vi "GetDriverFileName.vi"(11 "input string":string) -> (1 "DriverFileName":string, 2 "数组":string[](array[string]), 3 "子字符串之前":string)   [LabVIEW 2018]
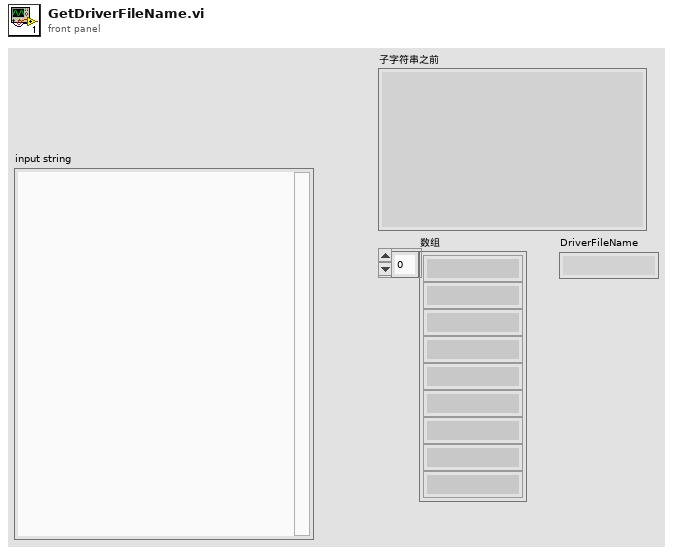
[diagram p1: front panel]
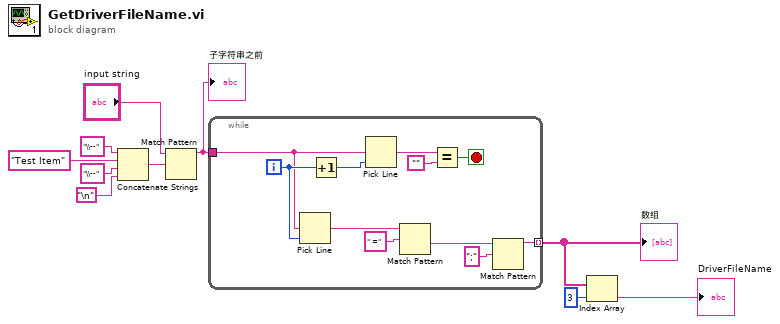
[diagram p0: block diagram]
diagram:
  n1 = Concatenate Strings("\\--" ("regular expression"), "Test Item" ("string"), "\\--" ("string"), "\n") -> (w5:string)
  n2 = Match Pattern(string="input string", regular expression=w5) -> (before substring=w4:string)  [unwired: 4 out]
  "子字符串之前" <- w4
  n3 = while {
    tunnel: w4 -> [w13]
    tunnel: [w11] -> w3 mode=indexing
    i -> [w14]
    stop <- w12 stop-if-true
    n4 = Pick Line(multi-line string=w13, line index=w14) -> (output string=w18:string)  [unwired: 1 out]
    n5 = Increment(x=w14) -> (x+1=w21:i32)
    n6 = Pick Line(multi-line string=w13, line index=w21) -> (output string=w20:string)  [unwired: 1 out]
    n7 = Match Pattern(string=w18, regular expression=" =") -> (after substring=w19:string)  [unwired: 4 out]
    n8 = Equal?(x=w20, y="") -> (x = y?=w12:bool)
    n9 = Match Pattern(string=w19, regular expression=";") -> (before substring=w11:string)  [unwired: 4 out]
  }
  "数组" <- w3
  n10 = Index Array(array=w3, index=3 ("索引")) -> (element=→"DriverFileName":string)
